vi "Clipped_Hist_Check.vi"(1 "Histogram Array":dbl[][](array[numeric]) format="%.2f") -> (0 "Error String":string)   [LabVIEW 2010]
uses:
  Globals/Meas_global.vi
  Globals/LDA_meas_global_1.vi
  Globals/LDA_meas_global_2.vi
panel:
  out "Max Vel":dbl=1.8339999999999999 format="%.2f"
  out "Min Vel":dbl=-1.8339999999999999 format="%.2f"
  out "Hist Index":i32
  out "Underflows":dbl format="%.2f"
  out "OverFlows":dbl format="%.2f"
  out "Instument Name":string
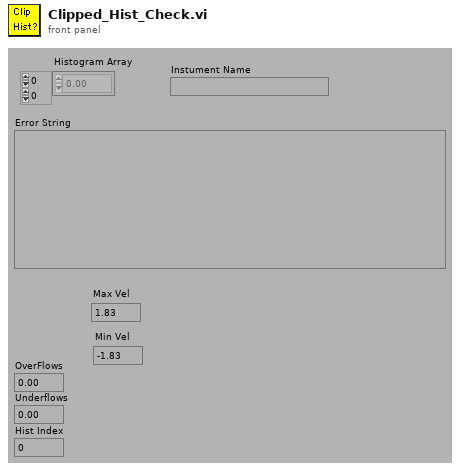
[diagram p1: front panel]
types:
  T1 = typedef "Analysis_info_cluster.ctl" = cluster{"Colour":u32, "Inst type":T2, "Inst name":string, "Symbol":string, "Code name":string, "Extra Info":string, "Inst Array":T3, "Index":i32, "Voltage Index":i32, "Extra Titles":string[], "Extra Values":string[]}
  T2 = typedef "Inst_type.ctl" = enum16{"Propeller anemometer", "Raw voltage", "Pressure Transducer", "Pitot-static tube", "Preston tube", "Hot wire", "Cross wire 1", "Cross wire 2", "Generic Linear", "Generic Polynomial", "Generic BackPoly", "Fast FID", "Thermocouple", "Cold wire", "Pulsed Wire", "LDA Vel", "LDA Tran time", "LDA Arr time"}
  T3 = typedef "Instrument_Array.ctl" = enum16{"PWA", "LDA", "Analogue"}
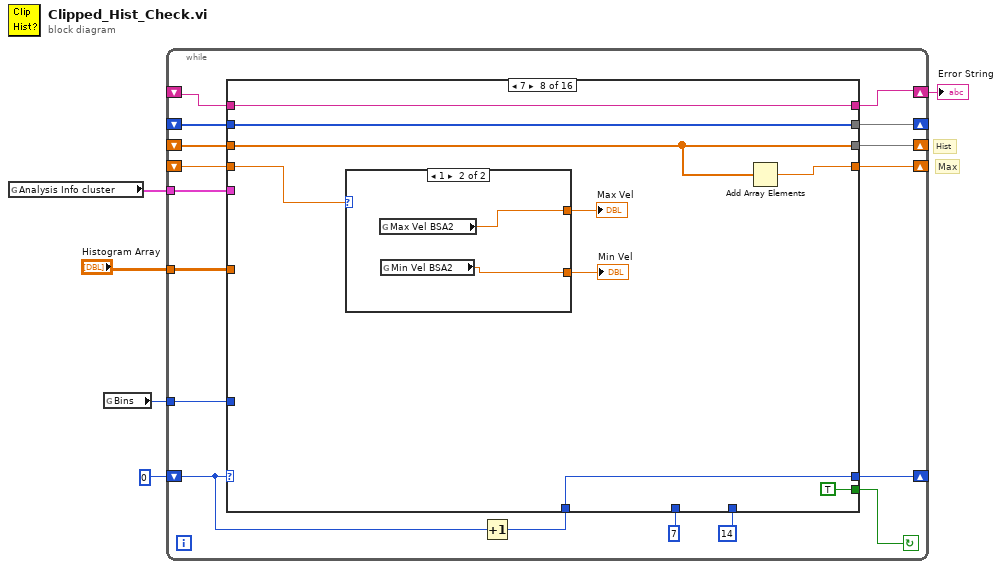
[diagram p0: block diagram]
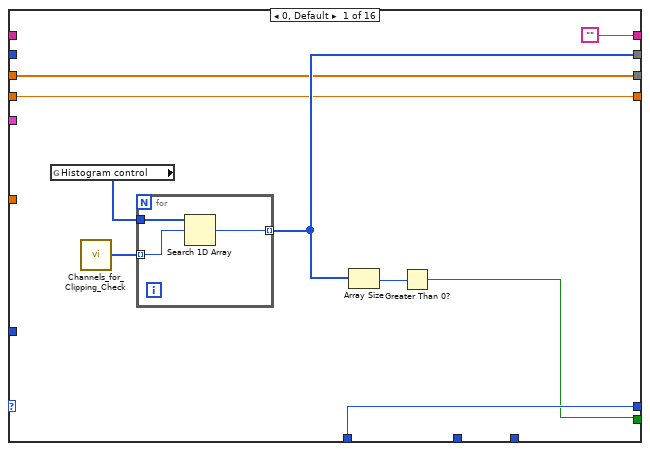
[diagram p2: hidden frame]
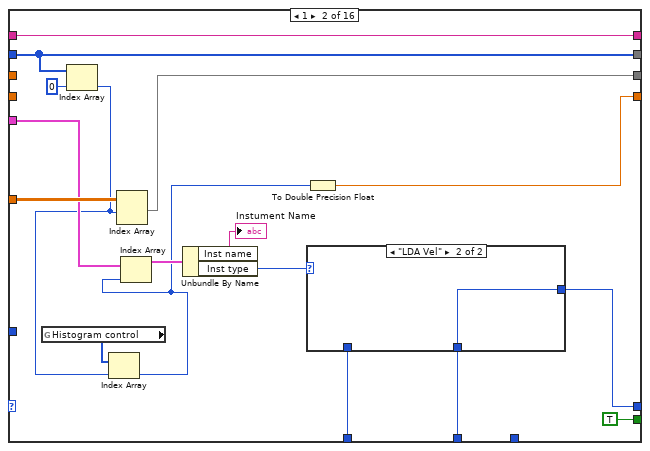
[diagram p3: hidden frame]
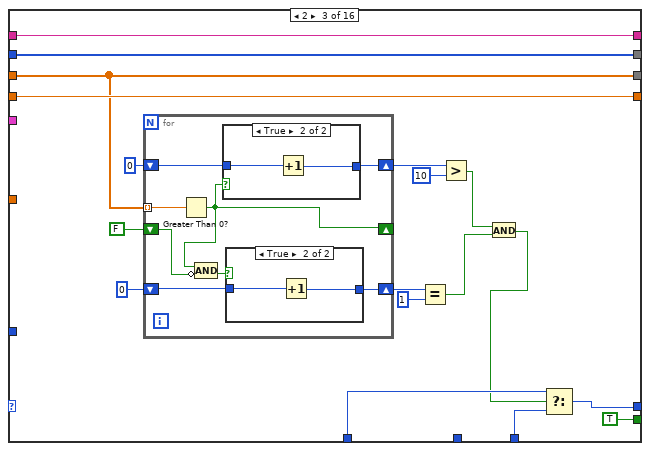
[diagram p5: hidden frame]
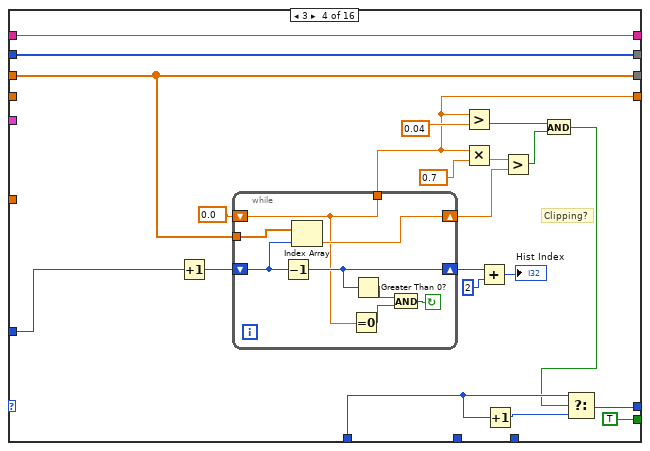
[diagram p8: hidden frame]
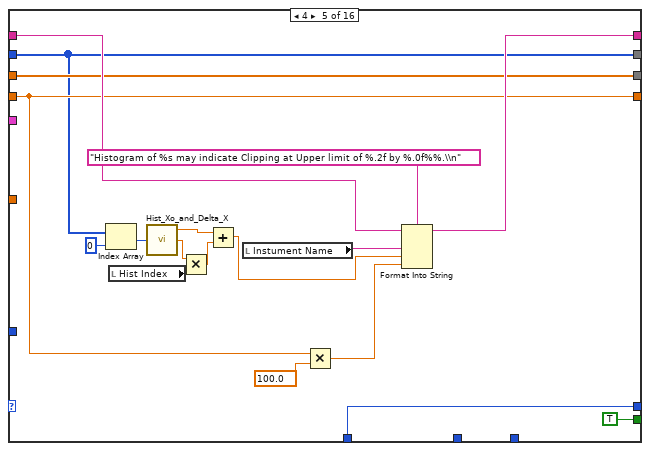
[diagram p9: hidden frame]
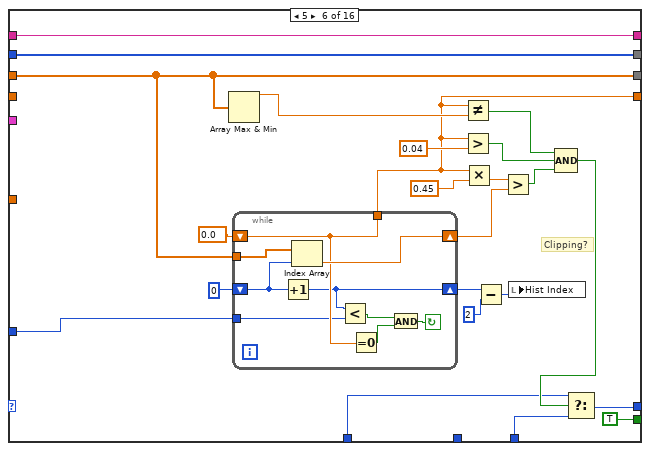
[diagram p10: hidden frame]
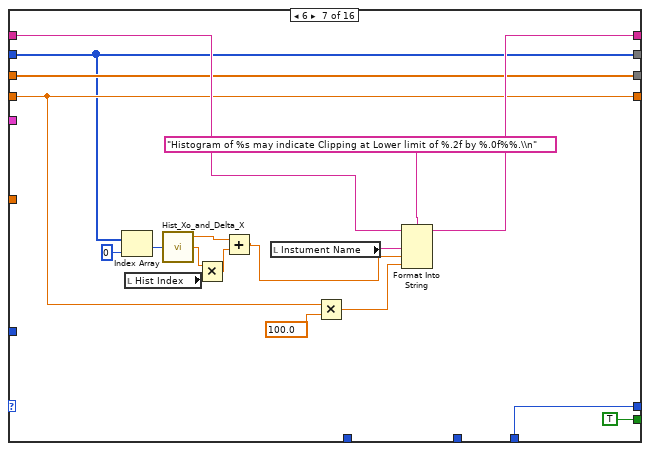
[diagram p11: hidden frame]
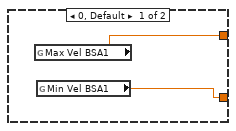
[diagram p12: hidden frame]
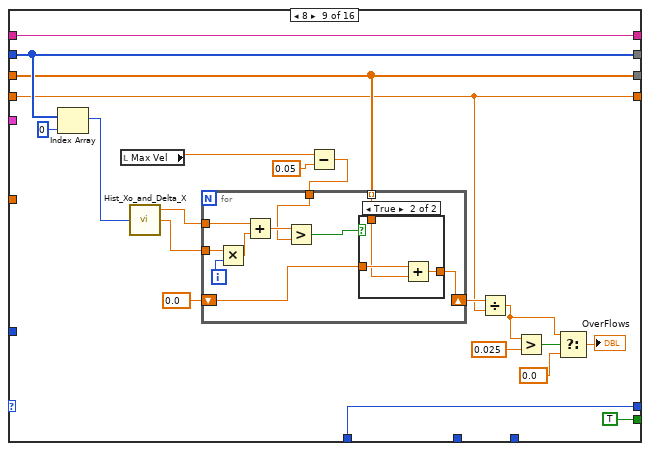
[diagram p13: hidden frame]
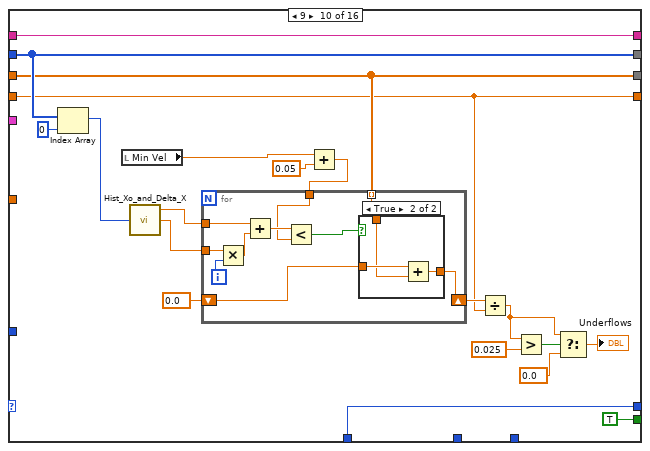
[diagram p15: hidden frame]
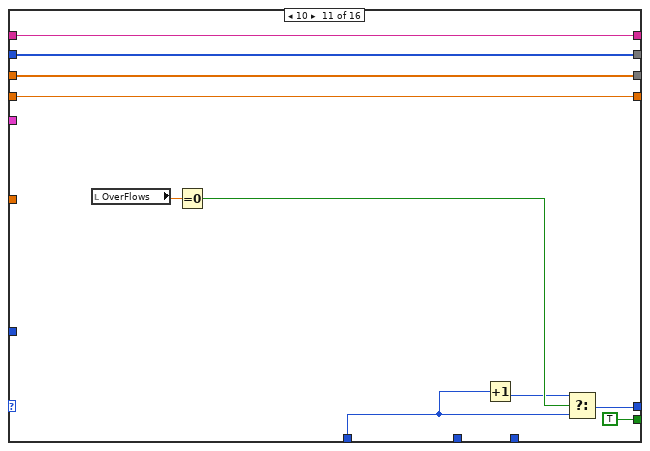
[diagram p17: hidden frame]
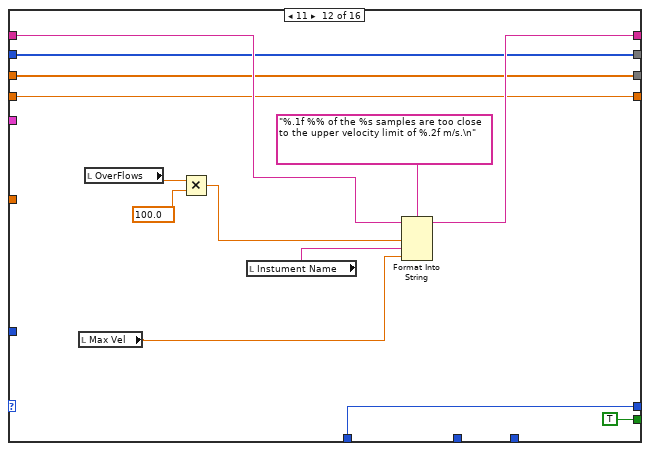
[diagram p18: hidden frame]
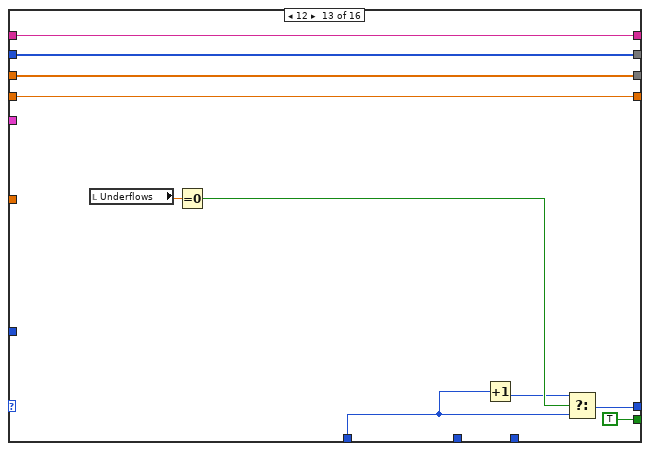
[diagram p19: hidden frame]
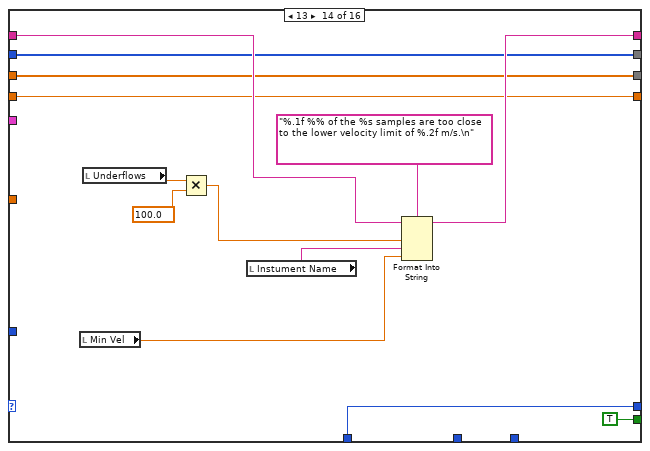
[diagram p20: hidden frame]
diagram:
  # "Max"
  # "Hist"
  n1 = global read "Meas_global.vi" "Analysis Info cluster"() -> (w1:T1[])
  n2 = global read "Meas_global.vi" "Bins"() -> (w2:i32)
  n3 = while {
    tunnel: w1 -> [w8]
    tunnel: w2 -> [w9]
    tunnel: "Histogram Array" -> [w10]
    shift-left: _ -> [w11]
    shift-right: [w13] -> _
    shift-left: _ -> [w12]
    shift-right: [w14] -> _
    shift-left: _ -> [w15]
    shift-right: [w16] -> w4
    shift-left: _ -> [w17]
    shift-right: [w18] -> _
    shift-left: 0 -> [w21]
    shift-right: [w19] -> _
    stop <- w22 continue-if-true
    n4 = Increment(x=w21) -> (x+1=w20:i32)
    n5 = case shown="7" w21 {
      tunnel: [w29 TRUE TRUE TRUE TRUE TRUE TRUE TRUE TRUE TRUE TRUE TRUE TRUE TRUE w312 FALSE] -> w22
      tunnel: w20 -> [w31 w42 w57 w98 w131 w142 _ w185 w201 w235 w265 w285 w288 w308 w314 w333]
      tunnel: [w31 w43 w55 w101 w131 w151 w177 w185 w201 w235 w267 w285 w290 w308 w315 w333] -> w19
      tunnel: [w25 w49 w70 w100 w122 w150 w167 w187 w212 w246 w269 w281 w292 w304 w317 w332] -> w18
      tunnel: w17 -> [_ w49 w70 w100 w122 w150 w167 w187 w212 w246 w269 w281 w292 w304 w320 w332]
      tunnel: ["" w48 w69 w99 w129 w149 w180 w190 w214 w248 w272 w283 w295 w306 w313 w327] -> w16
      tunnel: w15 -> [_ w48 w69 w99 w130 w149 w181 w190 w214 w248 w272 w284 w295 w307 w313 w327]
      tunnel: [w24 w35 w67 w91 w127 w139 w179 w189 w204 w238 w271 w282 w294 w305 w311 w331] -> w14
      tunnel: [w23 w40 w68 w89 w125 w137 w174 w186 w202 w236 w270 w276 w293 w299 w310 w330] -> w13
      tunnel: w12 -> [w24 _ w67 w91 w127 w139 w179 w189 w204 w238 w271 w282 w294 w305 w311 w331]
      tunnel: w11 -> [w23 _ w68 _ w125 _ w174 w188 w202 w236 w270 w276 w293 w299 w310 w330]
      tunnel: w10 -> [_ w47 _ _ _ _ _ _ _ _ _ _ _ _ _ _]
      tunnel: w9 -> [_ _ _ w92 _ w146 _ _ _ _ _ _ _ _ _ _]
      tunnel: w8 -> [_ w46 _ _ _ _ _ _ _ _ _ _ _ _ _ _]
      tunnel: 7 -> [_ w41 _ _ _ _ _ _ _ _ _ _ _ _ _ _]
      tunnel: 14 ("y") -> [_ _ w56 _ _ w141 w177 _ _ _ _ _ _ _ _ _]
      frame 0, Default {
        n6 = global read "Meas_global.vi" "Histogram control"() -> (w27:i32[])
        n7 = call "Channels_for_Clipping_Check.vi"() -> ("Channel Indicies"=w26:i32[])
        n8 = for {
          tunnel: w27 -> [w34]
          tunnel: w26 -> [w33] mode=indexing
          tunnel: [w32] -> w25 mode=indexing
          n9 = Search 1D Array(1D array=w34, element=w33) -> (index of element=w32:i32)  [unwired: 1 out]
        }
        n10 = Array Size(array=w25) -> (size(s)=w30:i32)
        n11 = Greater Than 0?(x=w30) -> (x > 0?=w29:bool)
      }
      frame 1 {
        n12 = global read "Meas_global.vi" "Histogram control"() -> (w39:i32[])
        n13 = Index Array(array=w49, index=0 ("Index")) -> (element=w37:i32)
        n14 = Index Array(array=w39, index=w37) -> (element=w36:i32)
        n15 = Index Array(array=w47, index (row)=w37) -> (element=w35:dbl[])  [unwired: 1 in]
        n16 = Index Array(array=w46, index=w36) -> (element=w45:T1)
        n17 = Unbundle By Name(w45) -> ("Inst name"=→"Instument Name":string, "Inst type"=w44:T2)
        n18 = case shown="\"LDA Vel\"" w44 {
          tunnel: [w52 w53] -> w43
          tunnel: w42 -> [w52 _]
          tunnel: w41 -> [_ w53]
          frame "Propeller anemometer", Default {
          }
          frame "LDA Vel" {
          }
        }
        n19 = To Double Precision Float(number=w36) -> (double precision float=w40:dbl)
      }
      frame 2 {
        n20 = for {
          tunnel: w67 -> [w79] mode=indexing
          shift-right: [w72] -> _
          shift-left: FALSE -> [w78]
          shift-right: [w75] -> w61
          shift-left: 0 -> [w76]
          shift-right: [w73] -> w63
          shift-left: 0 -> [w74]
          n21 = Greater Than 0?(x=w79) -> (x > 0?=w72:bool)
          n22 = Compound Arithmetic op=AND(w72, invert w78) -> (w77:bool)
          n23 = case shown="True" w72 {
            tunnel: w74 -> [w80 w82]
            tunnel: [w80 w81] -> w73
            frame False {
            }
            frame True {
              n24 = Increment(x=w82) -> (x+1=w81:i32)
            }
          }
          n25 = case shown="True" w77 {
            tunnel: w76 -> [w83 w85]
            tunnel: [w83 w84] -> w75
            frame False {
            }
            frame True {
              n26 = Increment(x=w85) -> (x+1=w84:i32)
            }
          }
        }
        n27 = Equal?(x=w61, y=1) -> (x = y?=w58:bool)
        n28 = Greater?(x=w63, y=10) -> (0:w59:bool)
        n29 = And(x=w59, y=w58) -> (x .and. y?=w54:bool)
        n30 = Select(t=w57, s=w54, f=w56) -> (s? t:f=w55:i32)
      }
      frame 3 {
        # "Clipping?"
        n31 = Increment(x=w92) -> (x+1=w106:i32)
        n32 = while {
          tunnel: [w107] -> w89
          tunnel: w91 -> [w114]
          shift-left: 0.0 -> [w107]
          shift-right: [w112] -> w103
          shift-left: w106 -> [w113]
          shift-right: [w111] -> w88
          stop <- w108 continue-if-true
          n33 = Decrement(x=w113) -> (x-1=w111:i32)
          n34 = Index Array(array=w114, index=w113) -> (element=w112:dbl)
          n35 = Equal To 0?(x=w107) -> (x = 0?=w109:bool)
          n36 = Greater Than 0?(x=w111) -> (x > 0?=w110:bool)
          n37 = And(x=w110, y=w109) -> (x .and. y?=w108:bool)
        }
        n38 = Greater?(x=w89, y=0.04) -> (0:w94:bool)
        n39 = Multiply(x=w89, y=0.7) -> (x*y=w104:dbl)
        n40 = Add(x=w88, y=2) -> (x+y=→"Hist Index":i32)
        n41 = Increment(x=w98) -> (x+1=w97:i32)
        n42 = Greater?(x=w104, y=w103) -> (0:w95:bool)
        n43 = And(x=w94, y=w95) -> (x .and. y?=w93:bool)
        n44 = Select(t=w98, s=w93, f=w97) -> (s? t:f=w101:i32)
      }
      frame 4 {
        n45 = Index Array(array=w122, index=0 ("Index")) -> (element=w121:i32)
        n46 = local read "Hist Index"() -> (w117:i32)
        n47 = call "Hist_Xo_and_Delta_X.vi"("Histogram index"=w121) -> ("Xo"=w119:dbl, "Delta X"=w118:dbl)  [unwired: 5 out]
        n48 = Multiply(x=w118, y=w117) -> (x*y=w120:dbl)
        n49 = Add(x=w119, y=w120) -> (x+y=w116:dbl)
        n50 = local read "Instument Name"() -> (w126:string)
        n51 = Multiply(x=w125, y=100.0) -> (x*y=w115:dbl)
        n52 = Format Into String(format string="Histogram of %s may indicate Clipping at Upper limit of %.2f by %.0f%%.\\n" ("Format String"), initial string=w130, w126, w116, w115) -> (resulting string=w129:string)  [unwired: 1 in, 1 out]
      }
      frame 5 {
        # "Clipping?"
        n53 = Array Max & Min(array=w139) -> (max value=w138:dbl)  [unwired: 3 out]
        n54 = while {
          tunnel: w146 -> [w157]
          tunnel: [w159] -> w137
          tunnel: w139 -> [w164]
          shift-left: 0.0 -> [w159]
          shift-right: [w162] -> w153
          shift-left: 0 -> [w163]
          shift-right: [w158] -> w135
          stop <- w160 continue-if-true
          n55 = Increment(x=w163) -> (x+1=w158:i32)
          n56 = Index Array(array=w164, index=w163) -> (element=w162:dbl)
          n57 = Less?(x=w158, y=w157) -> (x < y?=w156:bool)
          n58 = Equal To 0?(x=w159) -> (x = 0?=w161:bool)
          n59 = And(x=w156, y=w161) -> (x .and. y?=w160:bool)
        }
        n60 = Not Equal?(x=w137, y=w138) -> (x != y?=w136:bool)
        n61 = Greater?(x=w137, y=0.04) -> (0:w144:bool)
        n62 = Multiply(x=w137, y=0.45) -> (x*y=w154:dbl)
        n63 = Subtract(x=w135, y=2) -> (x-y=w134:i32)
        n64 = Greater?(x=w154, y=w153) -> (0:w145:bool)
        n65 = local write "Hist Index"(w134) -> ()
        n66 = Compound Arithmetic op=AND(w136, w144, w145) -> (w143:bool)
        n67 = Select(t=w142, s=w143, f=w141) -> (s? t:f=w151:i32)
      }
      frame 6 {
        n68 = Index Array(array=w167, index=0 ("Index")) -> (element=w172:i32)
        n69 = local read "Hist Index"() -> (w168:i32)
        n70 = call "Hist_Xo_and_Delta_X.vi"("Histogram index"=w172) -> ("Xo"=w170:dbl, "Delta X"=w169:dbl)  [unwired: 5 out]
        n71 = Multiply(x=w169, y=w168) -> (x*y=w171:dbl)
        n72 = Add(x=w170, y=w171) -> (x+y=w165:dbl)
        n73 = local read "Instument Name"() -> (w178:string)
        n74 = Multiply(x=w174, y=100.0) -> (x*y=w166:dbl)
        n75 = Format Into String(format string="Histogram of %s may indicate Clipping at Lower limit of %.2f by %.0f%%.\\n" ("Format String"), initial string=w181, w178, w165, w166) -> (resulting string=w180:string)  [unwired: 1 in, 1 out]
      }
      frame 7 {
        n76 = case shown="1" w188 {
          tunnel: [w193 w195] -> w184
          tunnel: [w192 w194] -> w183
          frame 0, Default {
            n77 = global read "LDA_meas_global_1.vi" "Max Vel BSA1"() -> (w193:dbl)
            n78 = global read "LDA_meas_global_1.vi" "Min Vel BSA1"() -> (w192:dbl)
          }
          frame 1 {
            n79 = global read "LDA_meas_global_2.vi" "Max Vel BSA2"() -> (w195:dbl)
            n80 = global read "LDA_meas_global_2.vi" "Min Vel BSA2"() -> (w194:dbl)
          }
        }
        "Min Vel" <- w183
        "Max Vel" <- w184
        n81 = Add Array Elements(numeric array=w189) -> (sum=w186:dbl)
      }
      frame 8 {
        n82 = Index Array(array=w212, index=0 ("Index")) -> (element=w206:i32)
        n83 = local read "Max Vel"() -> (w196:dbl)
        n84 = call "Hist_Xo_and_Delta_X.vi"("Histogram index"=w206) -> ("Xo"=w210:dbl, "Delta X"=w211:dbl)  [unwired: 5 out]
        n85 = Subtract(x=w196, y=0.05) -> (x-y=w209:dbl)
        n86 = for {
          tunnel: w211 -> [w224]
          tunnel: w210 -> [w223]
          tunnel: w209 -> [w218]
          shift-right: [w216] -> w203
          shift-left: 0.0 -> [w220]
          tunnel: w204 -> [w221] mode=indexing
          i -> [w225]
          n87 = Multiply(x=w224, y=w225) -> (x*y=w222:dbl)
          n88 = Add(x=w223, y=w222) -> (x+y=w219:dbl)
          n89 = Greater?(x=w219, y=w218) -> (0:w217:bool)
          n90 = case shown="True" w217 {
            tunnel: w221 -> [_ w228]
            tunnel: w220 -> [w226 w229]
            tunnel: [w226 w227] -> w216
            frame False {
            }
            frame True {
              n91 = Add(x=w229, y=w228) -> (x+y=w227:dbl)
            }
          }
        }
        n92 = Divide(x=w203, y=w202) -> (x/y=w199:dbl)
        n93 = Greater?(x=w199, y=0.025) -> (0:w200:bool)
        n94 = Select(t=w199, s=w200, f=0.0) -> (s? t:f=→"OverFlows":dbl)
      }
      frame 9 {
        n95 = Index Array(array=w246, index=0 ("Index")) -> (element=w240:i32)
        n96 = local read "Min Vel"() -> (w230:dbl)
        n97 = call "Hist_Xo_and_Delta_X.vi"("Histogram index"=w240) -> ("Xo"=w244:dbl, "Delta X"=w245:dbl)  [unwired: 5 out]
        n98 = Add(x=w230, y=0.05) -> (x+y=w243:dbl)
        n99 = for {
          tunnel: w245 -> [w258]
          tunnel: w244 -> [w257]
          tunnel: w243 -> [w252]
          shift-right: [w250] -> w237
          shift-left: 0.0 -> [w254]
          tunnel: w238 -> [w255] mode=indexing
          i -> [w259]
          n100 = Multiply(x=w258, y=w259) -> (x*y=w256:dbl)
          n101 = Add(x=w257, y=w256) -> (x+y=w253:dbl)
          n102 = Less?(x=w253, y=w252) -> (x < y?=w251:bool)
          n103 = case shown="True" w251 {
            tunnel: w255 -> [_ w262]
            tunnel: w254 -> [w260 w263]
            tunnel: [w260 w261] -> w250
            frame False {
            }
            frame True {
              n104 = Add(x=w263, y=w262) -> (x+y=w261:dbl)
            }
          }
        }
        n105 = Divide(x=w237, y=w236) -> (x/y=w233:dbl)
        n106 = Greater?(x=w233, y=0.025) -> (0:w234:bool)
        n107 = Select(t=w233, s=w234, f=0.0) -> (s? t:f=→"Underflows":dbl)
      }
      frame 10 {
        n108 = local read "OverFlows"() -> (w268:dbl)
        n109 = Equal To 0?(x=w268) -> (x = 0?=w266:bool)
        n110 = Increment(x=w265) -> (x+1=w264:i32)
        n111 = Select(t=w264, s=w266, f=w265) -> (s? t:f=w267:i32)
      }
      frame 11 {
        n112 = local read "Max Vel"() -> (w274:dbl)
        n113 = local read "OverFlows"() -> (w275:dbl)
        n114 = Multiply(x=w275, y=100.0) -> (x*y=w277:dbl)
        n115 = local read "Instument Name"() -> (w280:string)
        n116 = Format Into String(format string="%.1f %% of the %s samples are too close to the upper velocity limit of %.2f m/s.\n" ("Format String"), initial string=w284, w277, w280, w274) -> (resulting string=w283:string)  [unwired: 1 in, 1 out]
      }
      frame 12 {
        n117 = local read "Underflows"() -> (w291:dbl)
        n118 = Equal To 0?(x=w291) -> (x = 0?=w289:bool)
        n119 = Increment(x=w288) -> (x+1=w287:i32)
        n120 = Select(t=w287, s=w289, f=w288) -> (s? t:f=w290:i32)
      }
      frame 13 {
        n121 = local read "Min Vel"() -> (w297:dbl)
        n122 = local read "Underflows"() -> (w298:dbl)
        n123 = Multiply(x=w298, y=100.0) -> (x*y=w300:dbl)
        n124 = local read "Instument Name"() -> (w303:string)
        n125 = Format Into String(format string="%.1f %% of the %s samples are too close to the lower velocity limit of %.2f m/s.\n" ("Format String"), initial string=w307, w300, w303, w297) -> (resulting string=w306:string)  [unwired: 1 in, 1 out]
      }
      frame 14 {
        n126 = Array Subset(array=w320, index=1 ("Array Index")) -> (w317:i32[])  [unwired: 1 in]
        n127 = Array Size(array=w317) -> (size(s)=w318:i32)
        n128 = Greater Than 0?(x=w318) -> (x > 0?=w316:bool)
        n129 = case shown="True" w316 {
          tunnel: [w321 1 ("t")] -> w315
          tunnel: w314 -> [w321 _]
          tunnel: w313 -> [w324 _]
          tunnel: [w322 TRUE] -> w312
          frame False {
            n130 = Empty String/Path?(string/path=w324) -> (empty?=w323:bool)
            n131 = Not(x=w323) -> (.not. x?=w322:bool)
          }
          frame True {
          }
        }
      }
      frame 15 {
        n132 = global read "Meas_global.vi" "Over/Under string"() -> (w329:string)
        n133 = Concatenate Strings(w329, w327) -> (w328:string)
        n134 = global write "Meas_global.vi" "Over/Under string"(w328) -> ()
      }
    }
  }
  "Error String" <- w4
